vi "eFGV - Set Cursor.vi"(6 "FGV State":T1, 8 "Error In":errorcluster, 11 "Cursor Busy":bool) -> (0 "Error Out":errorcluster, 2 "Event Set Cursor":refnum<user-event>, 3 "Cursor Busy?":bool)   [LabVIEW 2020]
uses:
  Control/State - eFGV.ctl
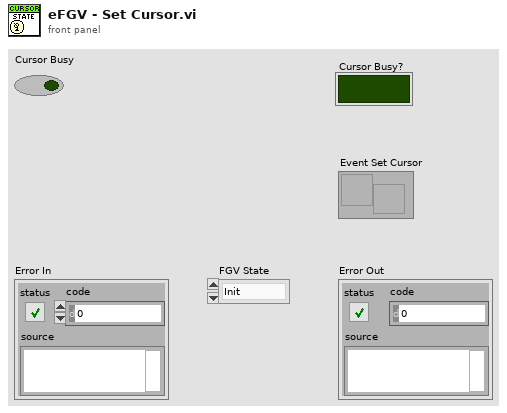
[diagram p1: front panel]
types:
  T1 = typedef "State - eFGV.ctl" = enum16{"Init", "Read", "Write", "Exit"}
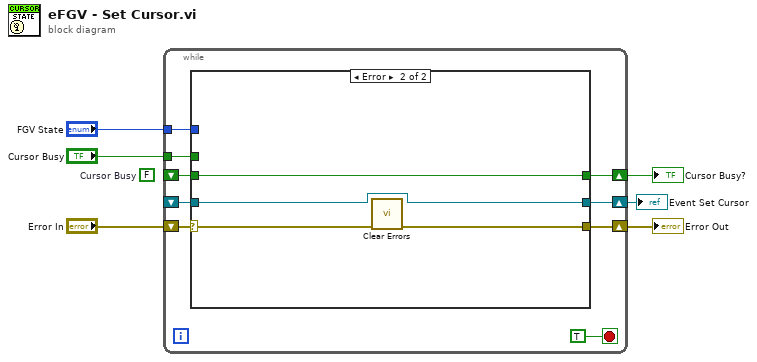
[diagram p0: block diagram]
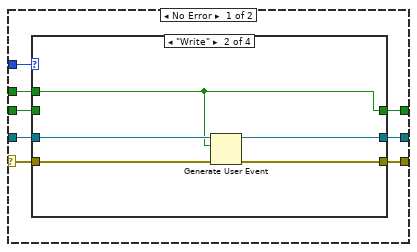
[diagram p2: hidden frame]
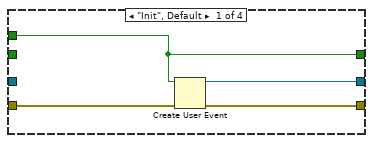
[diagram p3: hidden frame]
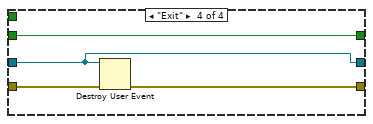
[diagram p5: hidden frame]
diagram:
  (unwired) FALSE  # Cursor Busy
  n1 = while {
    shift-right: [w14] -> w5
    shift-left: "Error In" -> [w15]
    tunnel: "FGV State" -> [w13]
    tunnel: "Cursor Busy" -> [w11]
    shift-right: [w10] -> w1
    shift-left: _ -> [w9]
    shift-right: [w7] -> w2
    shift-left: _ -> [w8]
    stop <- TRUE stop-if-true
    n2 = case shown="Error" w15 {
      selector: w15 -> [w23 w43]
      tunnel: w13 -> [w21 _]
      tunnel: w11 -> [w20 _]
      tunnel: [w22 w42] -> w14
      tunnel: [w19 w40] -> w10
      tunnel: w9 -> [w18 w40]
      tunnel: [w17 w41] -> w7
      tunnel: w8 -> [w16 w41]
      frame No Error {
        n3 = case shown="\"Write\"" w21 {
          tunnel: w20 -> [w24 w28 _ _]
          tunnel: w23 -> [w27 w32 w35 w39]
          tunnel: [w26 w31 w35 w38] -> w22
          tunnel: [w25 w29 w33 w37] -> w19
          tunnel: w18 -> [_ w30 w33 w37]
          tunnel: [w24 w28 w34 w36] -> w17
          tunnel: w16 -> [_ _ w34 w36]
          frame "Init", Default {
            n4 = Create User Event(user event datatype=w24, error in=w27) -> (user event=w25:refnum<user-event>, error out=w26:errorcluster)
          }
          frame "Write" {
            n5 = Generate User Event(user event=w30, event data cluster=w28, error in=w32) -> (user event out=w29:refnum<user-event>, error out=w31:errorcluster)  [unwired: 1 in]
          }
          frame "Read" {
          }
          frame "Exit" {
            n6 = Destroy User Event(user event=w37, error in=w39) -> (error out=w38:errorcluster)
          }
        }
      }
      frame Error {
        n7 = call <vilib>:"Clear Errors.vi"("error in (no error)"=w43) -> ("error out"=w42:errorcluster)  [unwired: 5 in, 1 out]
      }
    }
  }
  "Cursor Busy?" <- w2
  "Error Out" <- w5
  "Event Set Cursor" <- w1
